vi "Taking cells.vi"   [LabVIEW 2016]
types:
  T1 = typedef "LVHSConnector.ctl" = refnum<class "BrickReference.lvclass">
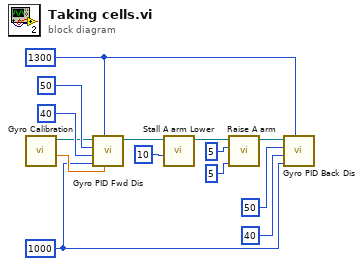
[diagram p0: block diagram]
diagram:
  w3 = 1000 ("Threshold to slow")
  w4 = 1300 ("Threshold to stop")
  n1 = call "Gyro Calibration.vi"() -> ("Degrees"=w11:sgl, "NXT/EV3"=w12:T1)  [unwired: 7 in, 1 out]
  n2 = call "Gyro PID Fwd Dis.vi"("Target angle"=w11, "Threshold to stop"=w4, "Threshold to slow"=w3, "Min. speed"=40, "Max. speed"=50, "EV3 in"=w12) -> ("EV3 out"=w10:T1)  [unwired: 5 in]
  n3 = call "Stall A arm Lower.vi"("Power"=i8 10, "NXT/EV3"=w10) -> ("NXT/EV3"=w8:T1)  [unwired: 9 in]
  n4 = call "Raise A arm.vi"("Power"=i8 5, "Rotation"=5, "EV3 in"=w8) -> ("EV3 out"=w5:T1)  [unwired: 8 in]
  n5 = call "Gyro PID Back Dis.vi"("Threshold to stop"=w4, "Threshold to slow"=w3, "Min. speed"=40, "Max. speed"=50, "EV3 in"=w5) -> ()  [unwired: 6 in, 1 out]
